vi "Temp Monitor start.vi"() -> ()   [LabVIEW 2019]
doc: "This is the Main VI for the temperature measurement of a thermistor.\n\nPaul K Dixon\nP3600\nCSUSB Physics"
uses:
  components/typedefs/exp sequence.ctl
  components/typedefs/PID exec cluster.ctl
  components/typedefs/temp mode enum.ctl
  components/globals/Bug man temp globals.vi
panel:
  out "Temp":dbl
  out "Temperature Graph":cluster{"t hist":dbl[], "T hist":dbl[]}(graph)
  out "exit loc":bool
  out "Exp Seq":T1 caption="Experimental Sequence"
  in  "proceed":bool
  in  "exit":bool
  in  "exit":bool
  out "Total elapsed time (s)":i32=10
  out "meas index":i32
  # "Thermistor\nTemperature\nMonitor"
  # "Paul K Dixon     \nP3600    \nCSUSB Physics"
  # "Note: This TAB is under system control"
  # "Experiment \nCompleted"
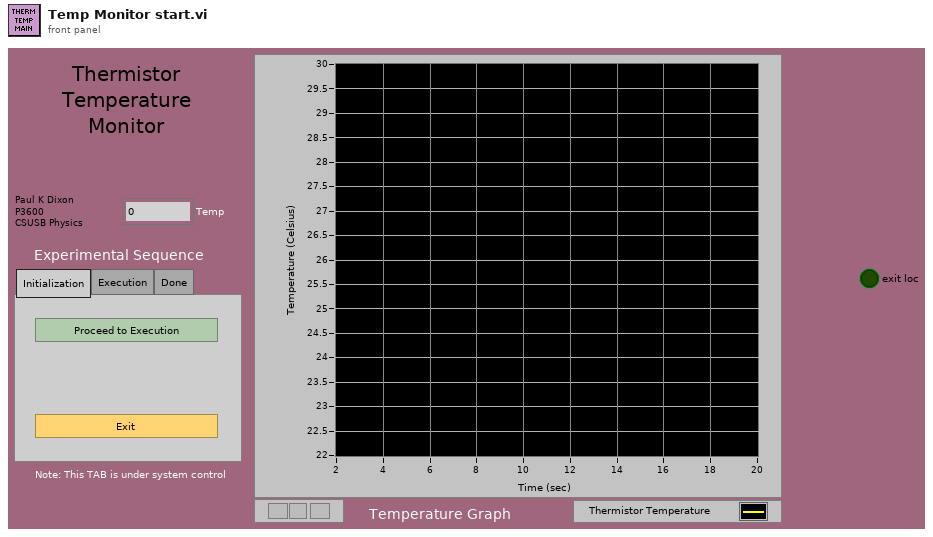
[diagram p1: front panel]
types:
  T1 = typedef "exp sequence.ctl" = enum32{"Initialization", "Execution", "Done"}
  T2 = typedef "temp mode enum.ctl" = enum16{"Setting up", "Listening to exec", "Exit"}
  T3 = typedef "PID exec cluster.ctl" = cluster{"error":errorcluster, "elapsed time (s)":dbl}
  T4 = typedef "temp cont cluster.ctl" = cluster{"exec":T5, "T status":T6, "utility":T7}
  T5 = typedef "temp exec cluster.ctl" = cluster{"T mode":T2, "log":bool, "thermistor":enum16{"solo", "bug"}}
  T6 = typedef "temp indicator.ctl" = cluster{"Temp":dbl}
  T7 = typedef "temp cont utility.ctl" = cluster{"meas index":i32, "wait (ms)":i32, "therm volt":dbl, "t T hist":dbl[][]}
  T8 = typedef "DAQ T state cluster.ctl" = cluster{"DAQ state":T9, "device":tag, "start (ms)":i32, "error":errorcluster, "T cont":T4}
  T9 = typedef "DAQ T state enum.ctl" = enum16{"Global comm", "Meas T ", "Wait", "Exit"}
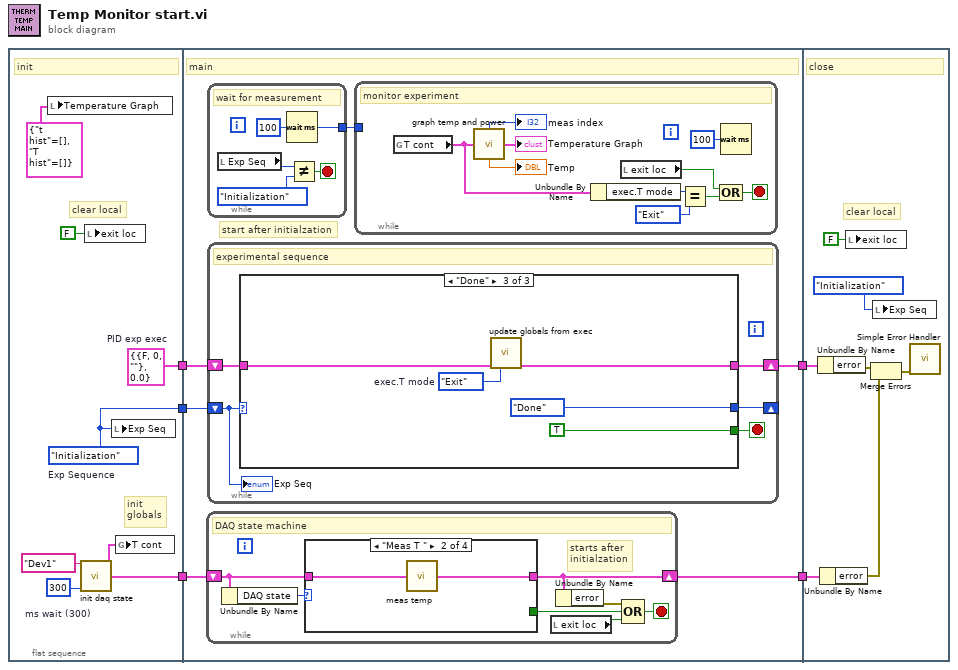
[diagram p0: block diagram]
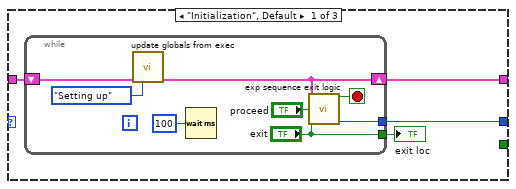
[diagram p2: hidden frame]
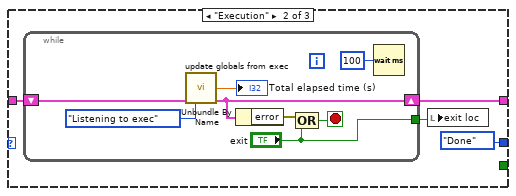
[diagram p3: hidden frame]
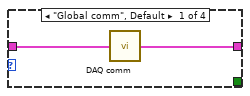
[diagram p4: hidden frame]
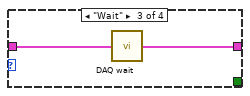
[diagram p5: hidden frame]
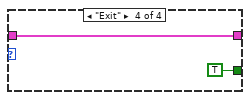
[diagram p6: hidden frame]
diagram:
  n1 = flat-sequence {
    tunnel: [w12] -> w3
    tunnel: [w10] -> w2
    tunnel: [w8] -> w1
    tunnel: [w19] -> w5
    tunnel: [w14] -> w4
    tunnel: w3 -> [w17]
    tunnel: w2 -> [w16]
    tunnel: w1 -> [w18]
    tunnel: w5 -> [w87]
    tunnel: w4 -> [w86]
    frame #0 {
      w12 = T3 {"error"={"status"=FALSE, "code"=0, "source"=""}, "elapsed time (s)"=0.0}  # PID exp exec
      w10 = exp_sequence."Initialization"  # Exp Sequence
      w13 = 300  # ms wait (300)
      # "clear local"
      # "init\nglobals"
      # "init"
      n2 = local write "Temperature Graph"(cluster{"t hist":dbl[], "T hist":dbl[]} {"t hist"=[], "T hist"=[]} ("Temperature Graph")) -> ()
      n3 = call "init daq state.vi"("device"=tag "Dev1", "T cont wait time (ms)"=w13) -> ("T cont out for global update"=w9:T4, "DAQ state start out"=w8:T8)  [unwired: 12 in]
      n4 = local write "exit loc"(FALSE ("exit")) -> ()
      n5 = local write "Exp Seq"(w10) -> ()
      n6 = global write "Bug man temp globals.vi" "T cont"(w9) -> ()
    }
    frame #1 {
      # "start after initialzation"
      # "main"
      n7 = while {
        shift-right: [w70] -> w14
        shift-left: w18 -> [w71]
        stop <- w74 stop-if-true
        # "starts after \ninitialzation"
        # "DAQ state machine"
        n8 = Unbundle By Name(w71) -> ("DAQ state"=w72:T9)
        n9 = case shown="\"Meas T \"" w72 {
          tunnel: [_ _ _ TRUE] -> w73
          tunnel: w71 -> [w77 w79 w81 w82]
          tunnel: [w76 w78 w80 w82] -> w70
          frame "Global comm", Default {
            n10 = call "DAQ comm.vi"("DAQ T state cluster in"=w77) -> ("DAQ T state cluster out"=w76:T8)  [unwired: 14 in]
          }
          frame "Meas T " {
            n11 = call "meas temp.vi"("DAQ state cluster in"=w79) -> ("DAQ state cluster out"=w78:T8)  [unwired: 14 in]
          }
          frame "Wait" {
            n12 = call "DAQ wait.vi"("DAQ state cluster in"=w81) -> ("DAQ state cluster out"=w80:T8)  [unwired: 14 in]
          }
          frame "Exit" {
          }
        }
        n13 = local read "exit loc"() -> (w69:bool)
        n14 = Unbundle By Name(w70) -> ("error"=w75:errorcluster)
        n15 = Compound Arithmetic op=OR(w75, w73, w69) -> (w74:bool)
      }
      n16 = while {
        tunnel: [w20] -> w15
        stop <- w21 stop-if-true
        # "wait for measurement"
        n17 = local read "Exp Seq"() -> (w23:T1)
        n18 = Wait (ms)(milliseconds to wait=u32 100) -> (millisecond timer value=w20:u32)
        n19 = Not Equal?(x=w23, y=exp_sequence."Initialization" ("Experimental Sequence")) -> (x != y?=w21:bool)
      }
      n20 = while {
        shift-right: [w36] -> _
        shift-left: w16 -> [w37]
        shift-right: [w38] -> w19
        shift-left: w17 -> [w39]
        stop <- w35 stop-if-true
        # "experimental sequence"
        n21 = case shown="\"Done\"" w37 {
          tunnel: w39 -> [w42 w55 w66]
          tunnel: [w43 w54 w65] -> w38
          tunnel: [w41 exp_sequence."Done" ("Experimental Sequence") exp_sequence."Done" ("Experimental Sequence")] -> w36
          tunnel: [_ _ TRUE] -> w35
          frame "Initialization", Default {
            n22 = while {
              shift-right: [w46] -> w43
              shift-left: w42 -> [w44]
              tunnel: [w48] -> w41
              tunnel: ["exit"] -> w40
              stop <- w49 stop-if-true
              n23 = call "update globals from exec.vi"("PID exp exec"=w44, "exec.T mode"=temp_mode_enum."Setting up") -> ("PID exp exec out"=w46:T3)  [unwired: 12 in, 1 out]
              n24 = Wait (ms)(milliseconds to wait=u32 100) -> ()  [unwired: 1 out]
              n25 = call "exp sequence exit logic.vi"("PID exp exec in"=w46, "proceed"="proceed", "exit"="exit") -> ("stop loop"=w49:bool, "Experimental Sequence"=w48:T1)  [unwired: 11 in]
            }
            "exit loc" <- w40
          }
          frame "Execution" {
            n26 = while {
              shift-right: [w61] -> w54
              shift-left: w55 -> [w56]
              tunnel: ["exit"] -> w53
              stop <- w62 stop-if-true
              n27 = call "update globals from exec.vi"("PID exp exec"=w56, "exec.T mode"=temp_mode_enum."Listening to exec") -> ("Total elapsed time (s)"=→"Total elapsed time (s)":dbl, "PID exp exec out"=w61:T3)  [unwired: 12 in]
              n28 = Unbundle By Name(w61) -> ("error"=w63:errorcluster)
              n29 = Compound Arithmetic op=OR(w63, "exit") -> (w62:bool)
              n30 = Wait (ms)(milliseconds to wait=u32 100) -> ()  [unwired: 1 out]
            }
            n31 = local write "exit loc"(w53) -> ()
          }
          frame "Done" {
            w64 = temp_mode_enum."Exit"  # exec.T mode
            n32 = call "update globals from exec.vi"("PID exp exec"=w66, "exec.T mode"=w64) -> ("PID exp exec out"=w65:T3)  [unwired: 12 in, 1 out]
          }
        }
        "Exp Seq" <- w37
      }
      n33 = while {
        tunnel: w15 -> [_]
        stop <- w31 stop-if-true
        # "monitor experiment"
        n34 = global read "Bug man temp globals.vi" "T cont"() -> (w29:T4)
        n35 = call "graph temp and power.vi"("T cont"=w29) -> ("meas index"=→"meas index":i32, "T plot"=→"Temperature Graph":cluster{"t hist":dbl[], "T hist":dbl[]}, "T status.Temp"=→"Temp":dbl)  [unwired: 12 in]
        n36 = Unbundle By Name(w29) -> ("exec.T mode"=w30:T2)
        n37 = local read "exit loc"() -> (w28:bool)
        n38 = Equal?(x=w30, y=temp_mode_enum."Exit" ("exec.T mode")) -> (x = y?=w32:bool)
        n39 = Compound Arithmetic op=OR(w28, w32) -> (w31:bool)
        n40 = Wait (ms)(milliseconds to wait=u32 100) -> ()  [unwired: 1 out]
      }
    }
    frame #2 {
      # "clear local"
      # "close"
      n41 = Unbundle By Name(w87) -> ("error"=w90:errorcluster)
      n42 = Unbundle By Name(w86) -> ("error"=w89:errorcluster)
      n43 = local write "exit loc"(FALSE ("exit")) -> ()
      n44 = Merge Errors(w90, w89) -> (w88:errorcluster)
      n45 = local write "Exp Seq"(exp_sequence."Initialization" ("Exp Seq")) -> ()
      n46 = call <vilib>:"Simple Error Handler.vi"("error in (no error)"=w88) -> ()  [unwired: 4 in, 5 out]
    }
  }
